vi "HEWH Energy Reset Check.vi"(8 "error in (no error)":errorcluster, 10 "Input Data":dbl[][](array[numeric]), 11 "Test Start Index":i32) -> (0 "error out":errorcluster, 3 "Test Start Index  (Full Index) out":i32)   [LabVIEW 2023]
panel:
  out "min value":dbl
  out "Output Data":dbl[][](array[numeric])
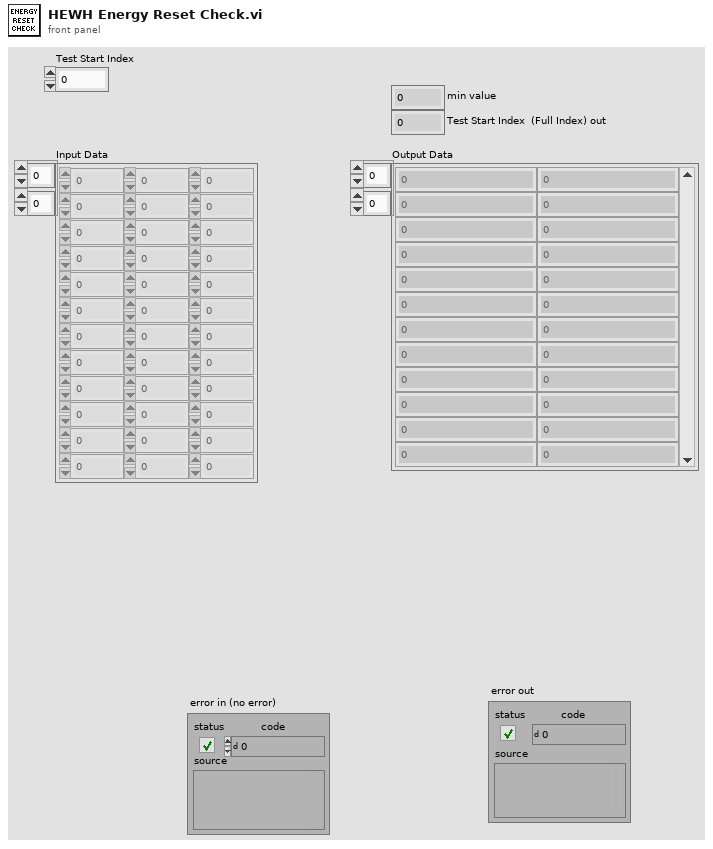
[diagram p1: front panel]
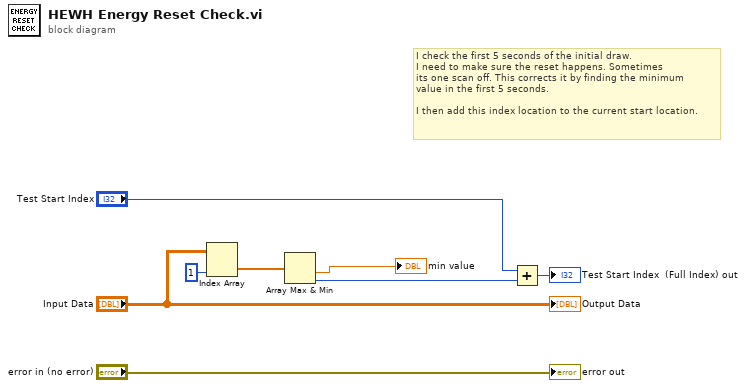
[diagram p0: block diagram]
diagram:
  # "I check the first 5 seconds of the initial draw. \nI need to make sure the reset happens. Sometimes\nits one scan off. This corrects it by finding the minimum\nvalue in the first 5 seconds.\n\nI then add this index location to the current start location."
  n1 = Index Array "Index Array"(array="Input Data", index (col)=1 ("disabled index (col)")) -> (element=w7:dbl[])  [unwired: 1 in]
  n2 = Array Max & Min(array=w7) -> (min value=→"min value":dbl, min index (indices)=w2:i32)  [unwired: 2 out]
  n3 = Add(x="Test Start Index", y=w2) -> (x+y=→"Test Start Index  (Full Index) out":i32)
  "Output Data" <- "Input Data"
  "error out" <- "error in (no error)"
